vi "ssh2_agent.vi"() -> ()   [LabVIEW 2013]
uses:
  libssh2/libssh2_agent_publickey_refnum.ctl
  libssh2/libssh2_init_default.vi
  libssh2/libssh2_session_handshake_tcp.vi
  libssh2/libssh2.lvlib
panel:
  out "authenticated":bool
  in  "hostname":string="localhost"
  in  "username":string
  out "error out":errorcluster
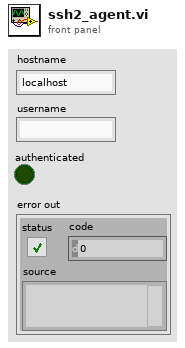
[diagram p1: front panel]
types:
  T1 = typedef "libssh2.lvlib/libssh2_agent_publickey_refnum.ctl" = refnum<k1>
  T2 = typedef "libssh2.lvlib/Session Refnum.ctl" = refnum<k1>
  T3 = typedef "libssh2.lvlib/Agent Refnum.ctl" = refnum<k1>
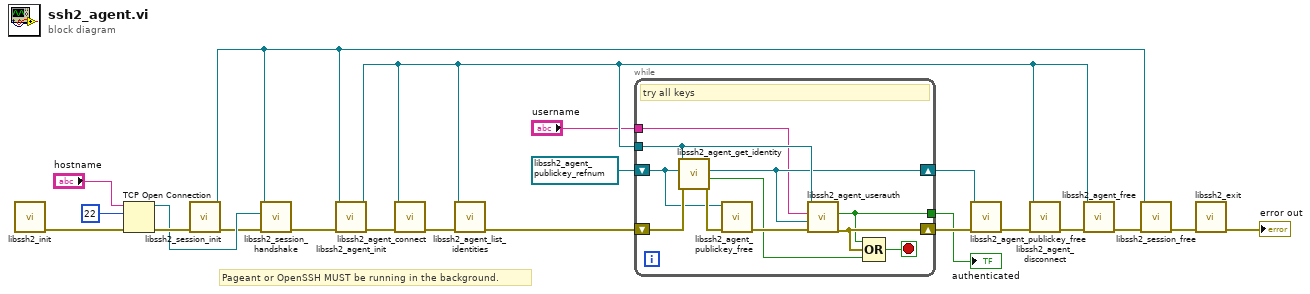
[diagram p0: block diagram]
diagram:
  w15 = T1 refnum items=["publickey"] ("store")
  # "Pageant or OpenSSH MUST be running in the background."
  n1 = call-poly "libssh2_init.vi"() -> ("error out"=w8:errorcluster)  [unwired: 11 in]
  n2 = TCP Open Connection(address="hostname", remote port or service name=u16 22, error in (no error)=w8) -> (connection ID=w6:refnum<k5>, error out=w7:errorcluster)  [unwired: 2 in]
  n3 = call "libssh2_session_init.vi"("error in (no error)"=w7) -> ("error out"=w5:errorcluster, "session"=w3:T2)  [unwired: 9 in]
  n4 = call-poly "libssh2_session_handshake.vi"("error in (no error)"=w5, "tcp connection"=w6, "session"=w3) -> ("error out"=w9:errorcluster)  [unwired: 8 in]
  n5 = call "libssh2_agent_init.vi"("error in (no error)"=w9, "session"=w3) -> ("error out"=w19:errorcluster, "agent"=w10:T3)  [unwired: 8 in]
  n6 = call "libssh2_agent_connect.vi"("error in (no error)"=w19, "agent"=w10) -> ("error out"=w17:errorcluster)  [unwired: 9 in]
  n7 = call "libssh2_agent_list_identities.vi"("error in (no error)"=w17, "agent"=w10) -> ("error out"=w16:errorcluster)  [unwired: 9 in]
  n8 = while {
    tunnel: w10 -> [w30]
    shift-right: [w29] -> w13
    shift-left: w15 -> [w31]
    shift-right: [w25] -> w14
    shift-left: w16 -> [w33]
    tunnel: "username" -> [w28]
    tunnel: [w23] -> w2
    stop <- w24 stop-if-true
    # "try all keys"
    n9 = call "libssh2_agent_get_identity.vi"("error in (no error)"=w33, "prev"=w31, "agent"=w30) -> ("error out"=w32:errorcluster, "end reached"=w26:bool, "store"=w29:T1)  [unwired: 6 in]
    n10 = call "libssh2_agent_publickey_free.vi"("error in (no error)"=w32, "public key"=w31) -> ("error out"=w27:errorcluster)  [unwired: 9 in]
    n11 = call "libssh2_agent_userauth.vi"("error in (no error)"=w27, "public key"=w29, "username"=w28, "agent"=w30) -> ("error out"=w25:errorcluster, "authenticated"=w23:bool)  [unwired: 6 in]
    n12 = Compound Arithmetic op=OR(w23, w25, w26) -> (w24:bool)
  }
  "authenticated" <- w2
  n13 = call "libssh2_agent_publickey_free.vi"("error in (no error)"=w14, "public key"=w13) -> ("error out"=w1:errorcluster)  [unwired: 9 in]
  n14 = call "libssh2_agent_disconnect.vi"("error in (no error)"=w1, "agent"=w10) -> ("error out"=w18:errorcluster)  [unwired: 9 in]
  n15 = call "libssh2_agent_free.vi"("error in (no error)"=w18, "agent"=w10) -> ("error out"=w22:errorcluster)  [unwired: 9 in]
  n16 = call "libssh2_session_free.vi"("error in (no error)"=w22, "session"=w3) -> ("error out"=w21:errorcluster)  [unwired: 9 in]
  n17 = call "libssh2_exit.vi"("error in (no error)"=w21) -> ("error out"=→"error out":errorcluster)  [unwired: 10 in]
